vi "Set Pixel Format.vi"(10 "Pixel Format":T1, 11 "IMAQdx Base Configure Strategy in":refnum<class "IMAQdx Base Configure Strategy.lvclass">) -> (3 "IMAQdx Base Configure Strategy out":refnum<class "IMAQdx Base Configure Strategy.lvclass">)   [LabVIEW 2024, in "IMAQdx Base Configure Strategy.lvclass"]
uses:
  IMAQdx Base Configure Strategy.lvclass
  IMAQdx Base Configure Strategy.lvclass/IMAQdx Base Configure Strategy.ctl
  Source/Typedefs/Generic Image/Pixel Format.ctl
  Source/Typedefs/Generic Image/Generic Image.lvclass
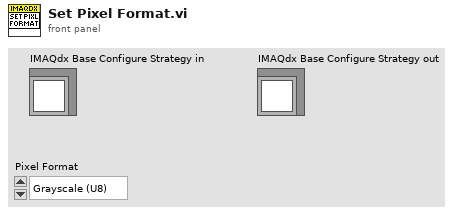
[diagram p1: front panel]
types:
  T1 = typedef "Generic Image.lvclass/Pixel Format.ctl" = enum16{"Grayscale (U8)", "Grayscale (I16)", "Grayscale (SGL)", "Complex (CSG)", "RGB (U32)", "HSL (U32)", "RGB (U64)", "Grayscale (U16)"}
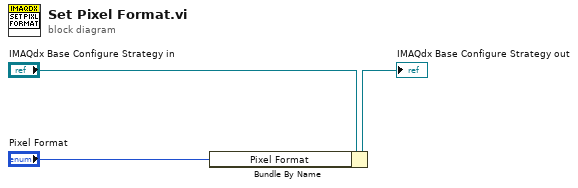
[diagram p0: block diagram]
diagram:
  n1 = Bundle By Name(cluster="IMAQdx Base Configure Strategy in", "Pixel Format"="Pixel Format") -> (→"IMAQdx Base Configure Strategy out":refnum<class "IMAQdx Base Configure Strategy.lvclass">)
